vi "ObstacleOurRadius.vi"(8 "Goal":dbl[](array[numeric]), 9 "Initial State":dbl[](array[numeric]), 10 "other robot":T1={"id"=0, "function"=enum."Attacker", "x"=0.0, "y"=0.0, "orientation"=0.0, "v_tangent"=0.0, "v_normal"=0.0, "v_ang"=0.0, "kick_x"=0.0, "kick_z"=0.0, "dribble"=FALSE, "Timestamp"=timestamp(0 s since 1904-01-01), "estimatives"={"est_v_tangent"=0.0, "est_v_normal"=0.0, "est_vx"=0.0, "est_vy"=0.0, "Pos Robot Est"=[]}, "dest_x_kick"=0.0, "dest_y_kick"=0.0, "Gap Coord"=[], "States"=enum."GoToTangent", "Path "=[], "Path  Smooth"=[], "Dest"=[], "vx_desired"=0.0, "vy_desired"=0.0, "slowBehavior"=FALSE, "VSSStates"=enum."Pass"}, 11 "Robot in":T1={"id"=0, "function"=enum."Attacker", "x"=0.0, "y"=0.0, "orientation"=0.0, "v_tangent"=0.0, "v_normal"=0.0, "v_ang"=0.0, "kick_x"=0.0, "kick_z"=0.0, "dribble"=FALSE, "Timestamp"=timestamp(0 s since 1904-01-01), "estimatives"={"est_v_tangent"=0.0, "est_v_normal"=0.0, "est_vx"=0.0, "est_vy"=0.0, "Pos Robot Est"=[]}, "dest_x_kick"=0.0, "dest_y_kick"=0.0, "Gap Coord"=[], "States"=enum."GoToTangent", "Path "=[], "Path  Smooth"=[], "Dest"=[], "vx_desired"=0.0, "vy_desired"=0.0, "slowBehavior"=FALSE, "VSSStates"=enum."Pass"}) -> (2 "obstacle enemy radius":dbl)   [LabVIEW 2020]
uses:
  Vision_class/Old vision/Controls/AI Robot.ctl
  Vision_class/Old vision/Controls/Functions Enum.ctl
  Vision_class/Old vision/Controls/AttackerStates.ctl
  Vision_class/Old vision/Controls/PathDests.ctl
  Vision_class/Old vision/Controls/PathDest.ctl
  Navigation/VSSNavigation/VSSAttackerStates.ctl
  <vilib>/Analysis/_algsub.llb/Real Vector Norm.vi
  <vilib>/Analysis/NI_AALPro.lvlib
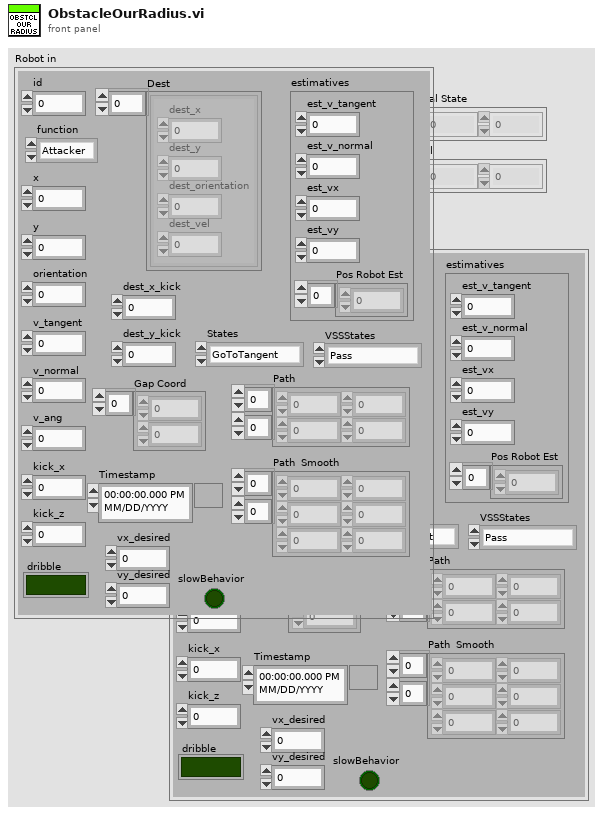
[diagram p1: front panel]
types:
  T1 = typedef "AI Robot.ctl" = cluster{"id":u32, "function":T2, "x":dbl, "y":dbl, "orientation":dbl, "v_tangent":dbl, "v_normal":dbl, "v_ang":dbl, "kick_x":dbl, "kick_z":dbl, "dribble":bool, "Timestamp":timestamp, "estimatives":cluster{"est_v_tangent":dbl, "est_v_normal":dbl, "est_vx":dbl, "est_vy":dbl, "Pos Robot Est":dbl[]}, "dest_x_kick":dbl, "dest_y_kick":dbl, "Gap Coord":dbl[], "States":T3, "Path ":dbl[][], "Path  Smooth":dbl[][], "Dest":T4, "vx_desired":dbl, "vy_desired":dbl, "slowBehavior":bool, "VSSStates":T6}
  T2 = typedef "Functions Enum.ctl" = enum16{"2nd Striker", "Attacker", "Goalie", "Defender", "Striker", "Goto 0", "Dummy", "Kicker", "ZigZag 0", "ZigZag 1", "ZigZag 2", "ZigZag 3", "ZigZag 4", "ZigZag 5", "ZigZag 6", "ZigZag 7", "ZigZag 8", ""}
  T3 = typedef "AttackerStates.ctl" = enum16{"Pass", "GoToTangent", "BallGetting", "GoToKick", ""}
  T4 = typedef "PathDests.ctl" = T5[]
  T5 = typedef "PathDest.ctl" = cluster{"dest_x":dbl, "dest_y":dbl, "dest_orientation":dbl, "dest_vel":dbl}
  T6 = typedef "VSSAttackerStates.ctl" = enum16{"Pass", "GoToTangent", "BallGetting", "GoToKick", "Rotate anti-clockwise", "Rotate Clockwise", ""}
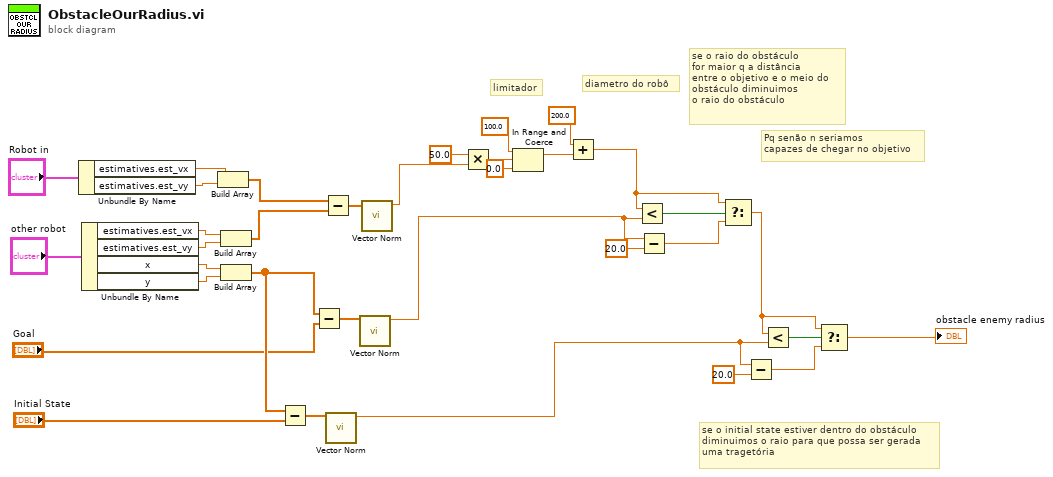
[diagram p0: block diagram]
diagram:
  # "limitador"
  # "diametro do robô"
  # "Pq senão n seriamos\ncapazes de chegar no objetivo"
  # "se o raio do obstáculo\nfor maior q a distância \nentre o objetivo e o meio do \nobstáculo diminuimos \no raio do obstáculo"
  # "se o initial state estiver dentro do obstáculo\ndiminuimos o raio para que possa ser gerada\numa tragetória"
  n1 = Unbundle By Name("Robot in") -> ("estimatives.est_vx"=w20:dbl, "estimatives.est_vy"=w19:dbl)
  n2 = Unbundle By Name("other robot") -> ("estimatives.est_vx"=w18:dbl, "estimatives.est_vy"=w17:dbl, "x"=w33:dbl, "y"=w32:dbl)
  n3 = Build Array(w20, w19) -> (w15:dbl[])
  n4 = Build Array(w18, w17) -> (w16:dbl[])
  n5 = Build Array(w33, w32) -> (w29:dbl[])
  n6 = Subtract(x=w29, y="Initial State") -> (x-y=w30:dbl[])
  n7 = Subtract(x=w29, y="Goal") -> (x-y=w31:dbl[])
  n8 = Subtract(x=w15, y=w16) -> (x-y=w14:dbl[])
  n9 = call-poly <vilib>:"Vector Norm.vi"("Input Vector"=w30) -> ("norm"=w24:dbl)  [unwired: 9 in, 1 out]
  n10 = call-poly <vilib>:"Vector Norm.vi"("Input Vector"=w31) -> ("norm"=w2:dbl)  [unwired: 9 in, 1 out]
  n11 = call-poly <vilib>:"Vector Norm.vi"("Input Vector"=w14) -> ("norm"=w3:dbl)  [unwired: 9 in, 1 out]
  n12 = Multiply(x=50.0, y=w3) -> (x*y=w12:dbl)
  n13 = In Range and Coerce(upper limit=100.0, x=w12, lower limit=0.0) -> (coerced(x)=w9:dbl)  [unwired: 1 out]
  n14 = Add(x=200.0, y=w9) -> (x+y=w6:dbl)
  n15 = Less?(x=w6, y=w2) -> (x < y?=w7:bool)
  n16 = Subtract(x=w2, y=20.0) -> (x-y=w4:dbl)
  n17 = Select(t=w6, s=w7, f=w4) -> (s? t:f=w1:dbl)
  n18 = Subtract(x=w24, y=20.0) -> (x-y=w23:dbl)
  n19 = Less?(x=w1, y=w24) -> (x < y?=w27:bool)
  n20 = Select(t=w1, s=w27, f=w23) -> (s? t:f=→"obstacle enemy radius":dbl)
